vi "Register Button Value Change Events.vi"(8 "error in (no error)":errorcluster, 10 "Button Event Refnum In":refnum<event-registration>, 11 "Panel Form Controller in":refnum<class "Panel Form Controller.lvclass">) -> (0 "error out":errorcluster, 2 "Button Event Refnum Out":refnum<event-registration>, 3 "Panel Form Controller out":refnum<class "Panel Form Controller.lvclass">)   [LabVIEW 2020, in "Panel Form Controller.lvlib" / "Panel Form Controller.lvclass"]
uses:
  Panel Form Controller.lvclass
  Panel Form Controller.lvclass/Panel Form Controller.ctl
  Button.lvclass/Button.ctl
  Button.lvclass
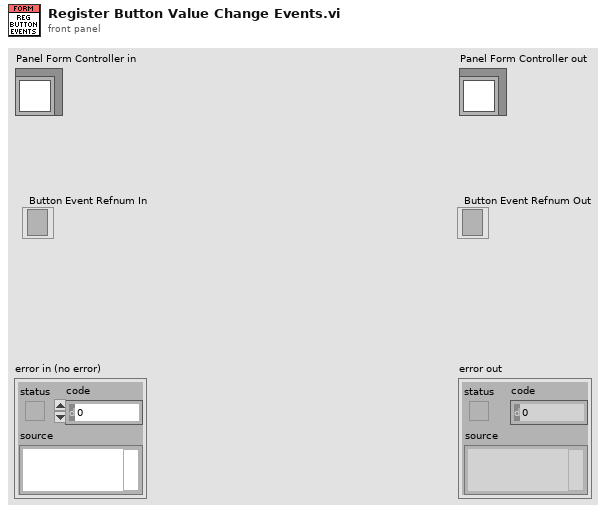
[diagram p1: front panel]
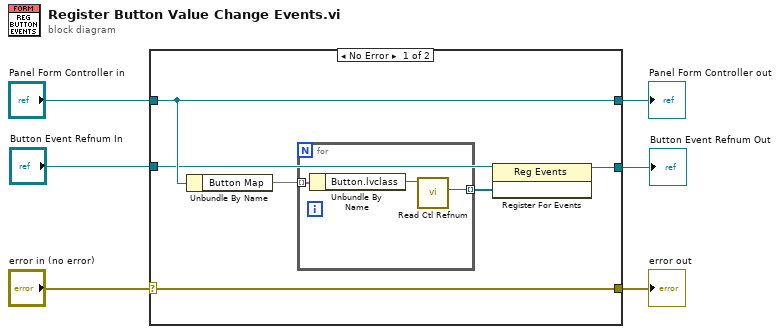
[diagram p0: block diagram]
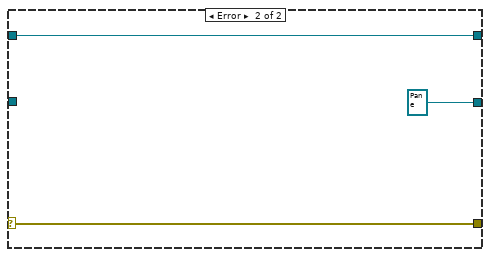
[diagram p2: hidden frame]
diagram:
  n1 = case shown="No Error" "error in (no error)" {
    selector: "error in (no error)" -> [w12 w18]
    tunnel: [w12 w18] -> w5
    tunnel: [w11 w17] -> w3
    tunnel: "Panel Form Controller in" -> [w11 w17]
    tunnel: [w9 refnum<event-registration> refnum ("field value change")] -> w2
    tunnel: "Button Event Refnum In" -> [w8 _]
    frame No Error {
      n2 = Unbundle By Name(w11) -> ("Button Map"=w10:map{string, refnum<class "Button.lvclass">})
      n3 = for {
        tunnel: w10 -> [w15] mode=indexing
        tunnel: [w13] -> w7 mode=indexing
        n4 = Unbundle By Name(w15) -> ("Button.lvclass"=w14:refnum<class "Button.lvclass">)
        n5 = call "Read Ctl Refnum.vi"("Button in"=w14) -> ("Ctl Refnum"=w13:refnum<vi>)  [unwired: 8 in, 2 out]
      }
      n6 = register-events(reference=w8, w7) -> (reference out=w9:refnum<event-registration>)  [unwired: 1 in, 1 out]
    }
    frame Error {
    }
  }
  "error out" <- w5
  "Panel Form Controller out" <- w3
  "Button Event Refnum Out" <- w2
